vi "BotSpeakSerial_Init.vi"(3 "Connection In":T1) -> (0 "error out":errorcluster, 1 "Connection out":T1)   [LabVIEW 2012]
uses:
  <userlib>/BotSpeak/VIs/SubVIs/CommState.ctl
  <userlib>/BotSpeak/VIs/Direct/BotSpeak_Control.ctl
  <vilib>/Instr/_visa.llb/VISA Configure Serial Port (Instr).vi
  <userlib>/BotSpeak/VIs/SubVIs/BotSpeak_Globals.vi
panel:
  out "Init?":bool
  out "Address":string
  out "VISA resource name out":refnum<visa-resource-name>
  out "StartupWait":i32
  out "Com Protocol":string
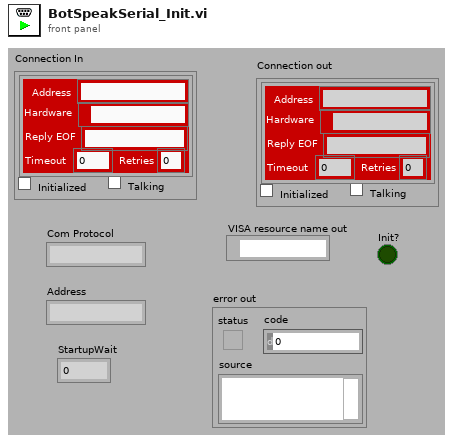
[diagram p1: front panel]
types:
  T1 = typedef "CommState.ctl" = cluster{"Bot Settings":T2, "Initialized":bool, "Talking":bool}
  T2 = typedef "BotSpeak_Control.ctl" = cluster{"Address":string, "Reply EOF":string, "Hardware":path, "Retries":i8, "Timeout":i32}
  T3 = typedef "BotSpeak.HardwareSpecs.ctl" = cluster{"Hardware Name":string, "Hardware URL":string, "ComType":enum16{"Undefined", "Serial", "TCPIP", "Console"}, "TCP Port":i32, "DefaultAddress":string, "Retries":i32, "Translate":enum16{"None", "Tiny", "URAPI"}, "MaxScriptSize":i32, "MaxVarNumber":i32, "StartupWait":i32, "Patience":i32, "Startup Patience":i32, "Hardware Help":string, "Com Protocol":string, "Translator":cluster{"BotSpeak CMD":string, "CMD out":string}[], "Init Code":string, "Variable Format":enum16{"INT", "FLOAT", "FIXED"}}
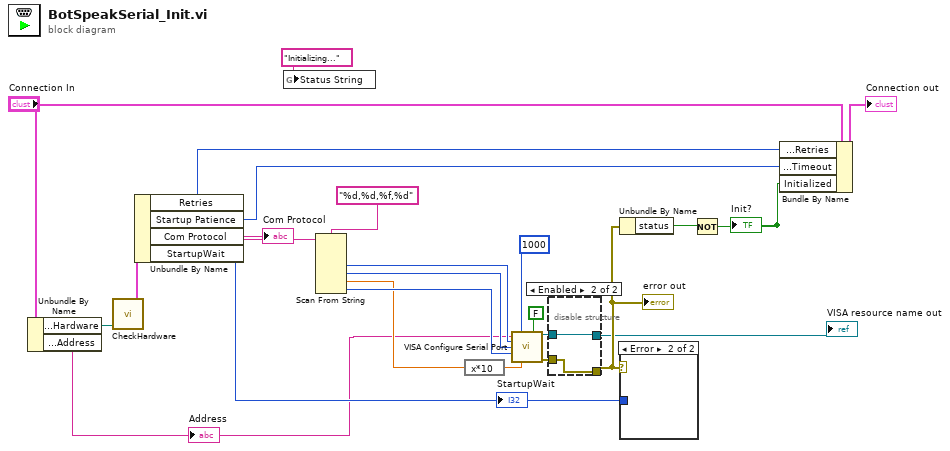
[diagram p0: block diagram]
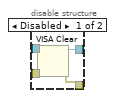
[diagram p2: hidden frame]
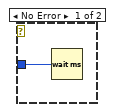
[diagram p3: hidden frame]
diagram:
  n1 = Unbundle By Name("Connection In") -> ("Bot Settings.Hardware"=w14:path, "Bot Settings.Address"=w1:string)
  "Address" <- w1
  n2 = call <userlib>:"CheckHardware.vi"("Hardware"=w14) -> ("HardwareSpecs"=w13:T3)  [unwired: 2 in]
  n3 = Unbundle By Name(w13) -> ("Retries"=w3:i32, "Startup Patience"=w4:i32, "Com Protocol"=w12:string, "StartupWait"=w11:i32)
  "Com Protocol" <- w12
  "StartupWait" <- w11
  n4 = global write "BotSpeak_Globals.vi" "Status String"("Initializing..." ("Status String")) -> ()
  n5 = Scan From String(format string="%d,%d,%f,%d", input string=w12) -> (output 1=w20:i32, output 2=w21:i32, output 3=w22:dbl, output 4=w23:i32)  [unwired: 6 in, 3 out]
  n6 = expression code="x*10"(w22) -> (w24:dbl)
  n7 = call-poly "VISA Configure Serial Port"("VISA resource name"=w1, "timeout (10sec)"=u32 1000, "Enable Termination\nChar (T)"=FALSE ("Enable Termination\nChar (T)"), "baud rate (9600)"=w20, "data bits (8)"=w21, "parity (0:none)"=w23, "stop bits (10: 1 bit)"=w24) -> ("VISA resource name out"=w15:refnum<visa-resource-name>, "error out"=w8:errorcluster)  [unwired: 7 in]
  n8 = disable-structure shown="Enabled" {
    disable-tunnel: w15 -> [w28 w29]
    disable-tunnel: w8 -> [w27 w30]
    disable-tunnel: [w26 w30] -> w7
    disable-tunnel: [w25 w29] -> w6
    frame Disabled {
      n9 = VISA Clear(VISA resource name=w28, error in (no error)=w27) -> (VISA resource name out=w25:refnum<visa-resource-name>, error out=w26:errorcluster)
    }
    frame Enabled {
    }
  }
  "error out" <- w7
  "VISA resource name out" <- w6
  n10 = Unbundle By Name(w7) -> ("status"=w18:bool)
  n11 = case shown="Error" w7 {
    tunnel: w11 -> [w31 _]
    frame No Error {
      n12 = Wait (ms)(milliseconds to wait=w31) -> ()  [unwired: 1 out]
    }
    frame Error {
    }
  }
  n13 = Not(x=w18) -> (.not. x?=w9:bool)
  "Init?" <- w9
  n14 = Bundle By Name(cluster="Connection In", "Bot Settings.Retries"=w3, "Bot Settings.Timeout"=w4, "Initialized"=w9) -> (→"Connection out":T1)
